vi "convert_voltage_to_opening.vi"(4 "bypass_valve_v0":dbl format="%#_13g", 6 "run_valve_v0":dbl format="%#_13g", 8 "status_in":bool, 10 "bypass_valve_voltage":dbl, 11 "run_valve_voltage":dbl) -> (0 "status_out":bool, 2 "bypass_valve_opening":dbl, 3 "run_valve_opening":dbl)   [LabVIEW 2019]
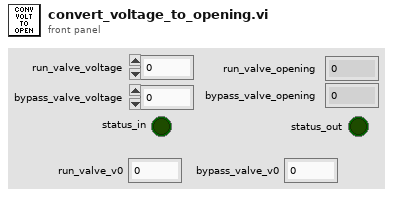
[diagram p1: front panel]
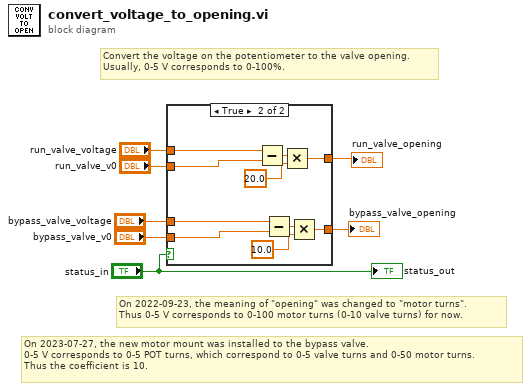
[diagram p0: block diagram]
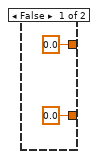
[diagram p2: hidden frame]
diagram:
  # "On 2023-07-27, the new motor mount was installed to the bypass valve.\n0-5 V corresponds to 0-5 POT turns, which correspond to 0-5 valve turns and 0-50 motor turns.\nThus the coefficient is 10."
  # "On 2022-09-23, the meaning of \"opening\" was changed to \"motor turns\".\nThus 0-5 V corresponds to 0-100 motor turns (0-10 valve turns) for now."
  # "Convert the voltage on the potentiometer to the valve opening.\nUsually, 0-5 V corresponds to 0-100%."
  n1 = case shown="True" "status_in" {
    tunnel: [0.0 w15] -> w7
    tunnel: [0.0 w14] -> w6
    tunnel: "run_valve_voltage" -> [_ w13]
    tunnel: "bypass_valve_voltage" -> [_ w11]
    tunnel: "run_valve_v0" -> [_ w12]
    tunnel: "bypass_valve_v0" -> [_ w10]
    frame False {
    }
    frame True {
      n2 = Subtract(x=w13, y=w12) -> (x-y=w19:dbl)
      n3 = Subtract(x=w11, y=w10) -> (x-y=w17:dbl)
      n4 = Multiply(x=w19, y=20.0) -> (x*y=w15:dbl)
      n5 = Multiply(x=w17, y=10.0) -> (x*y=w14:dbl)
    }
  }
  "run_valve_opening" <- w7
  "bypass_valve_opening" <- w6
  "status_out" <- "status_in"
